vi "ELVIS III v1.1 Open SPI.vi"(7 "Allow multiple opens?":bool, 8 "error in (no error)":errorcluster, 10 "Channel Name":string, 11 "Resource name":T1 caption="RIO Device") -> (0 "error out":errorcluster, 2 "SPI Channel":T2, 3 "myRIO Ref Out":T3)   [LabVIEW 2021]
uses:
  <vilib>/myRIO/Common/Instrument Driver Framework/Utilities/typedefs/myRIO v1.0 Reference.ctl
  <vilib>/myRIO/Common/Instrument Driver Framework/Utilities/typedefs/Generic FPGA Reference.ctl
  <vilib>/myRIO/Common/Instrument Driver Framework/myRIO v1.0/SPI/typedefs/SPI Channels Enum.ctl
  <vilib>/userDefined/High Color/nirio_resource_hc.ctl
  <vilib>/myRIO/Common/Instrument Driver Framework/ELVIS III v1.0/SPI/typedefs/ELVIS III v1.0 SPI Channels Enum.ctl
  <vilib>/myRIO/Common/Instrument Driver Framework/ELVIS III v1.0/SPI/vis/ELVIS III v1.0 Build MUX Configuration SPI.vi
  <vilib>/myRIO/Common/Instrument Driver Framework/ELVIS III v1.0/Resource Manager/vis/ELVIS III v1.0 Create Configuration List.vi
  <vilib>/Utility/VariantDataType/GetNumericInfo.vi
  <vilib>/Utility/error.llb/Error Cluster From Error Code.vi
  <vilib>/myRIO/Common/Instrument Driver Framework/ELVIS III v1.0/Resource Manager/vis/ELVIS III v1.0 Reserve Channel List.vi
  <vilib>/myRIO/Common/Instrument Driver Framework/ELVIS III v1.0/Resource Manager/vis/ELVIS III v1.0 Configure IO.vi
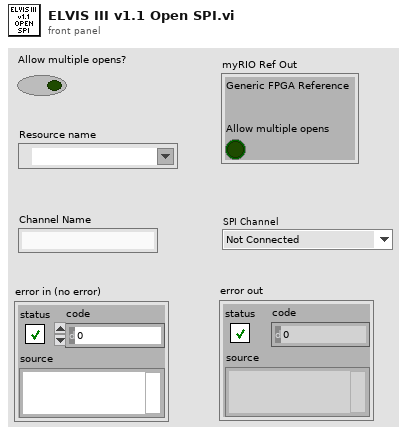
[diagram p1: front panel]
types:
  T1 = typedef "nirio_resource_hc.ctl" = tag
  T2 = typedef "SPI Channels Enum.ctl" = enum16{"Not Connected", "A/SPI", "B/SPI", "SPI/SPI"}
  T3 = typedef "myRIO v1.0 Reference.ctl" = cluster{"Generic FPGA Reference":T4, "Allow multiple opens":bool}
  T4 = typedef "Generic FPGA Reference.ctl" = refnum<k20>
  T5 = typedef "ELVIS III v1.0 SPI Channels Enum.ctl" = enum16{"Not Connected", "A/SPI", "B/SPI"}
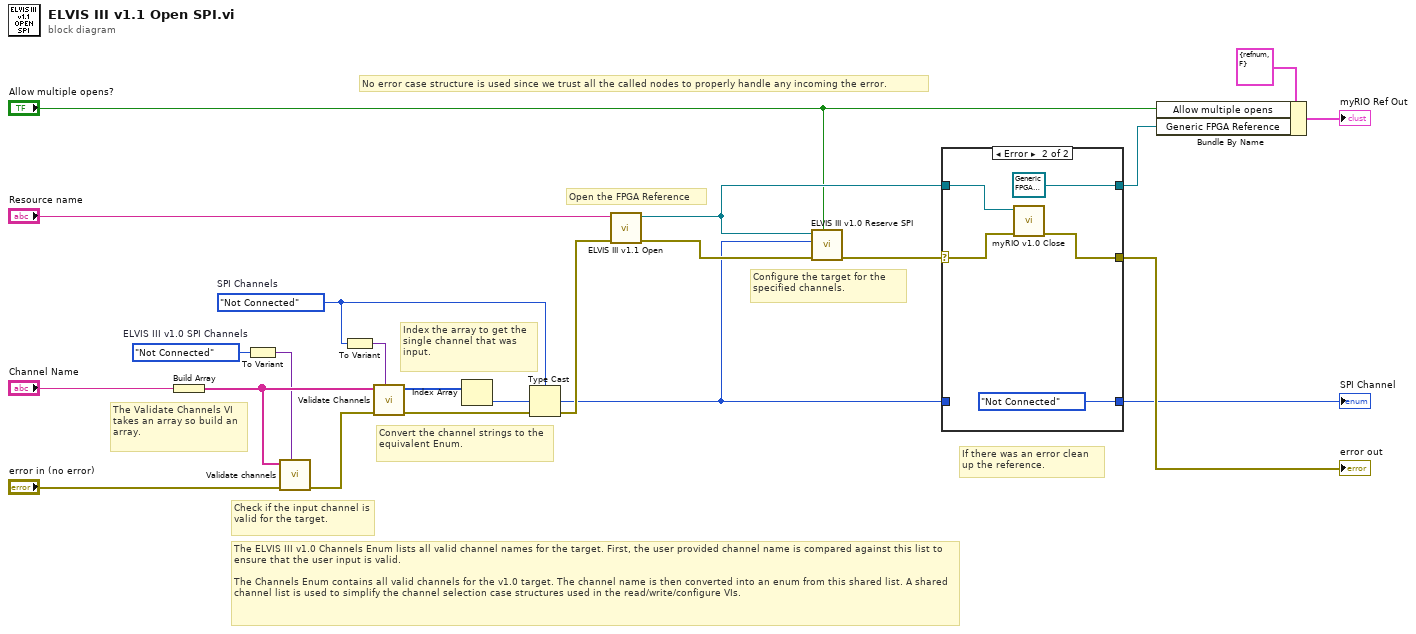
[diagram p0: block diagram]
diagram:
  w1 = SPI_Channels_Enum."Not Connected"  # SPI Channels
  w3 = ELVIS_III_v1.0_SPI_Channels_Enum."Not Connected"  # ELVIS III v1.0 SPI Channels
  # "The ELVIS III v1.0 Channels Enum lists all valid channel names for the target. First, the user provided channel name is compared against this list to ensure that the user input is valid.\n\nThe Channels Enum contains all valid channels for the v1.0 target. The channel name is then converted into an enum from this shared list. A shared channel list is used to simplify the channel selection case structures used in the read/write/configure VIs."
  # "Index the array to get the single channel that was input."
  # "The Validate Channels VI takes an array so build an array."
  # "If there was an error clean up the reference."
  # "Configure the target for the specified channels."
  # "Open the FPGA Reference"
  # "No error case structure is used since we trust all the called nodes to properly handle any incoming the error."
  # "Convert the channel strings to the equivalent Enum."
  # "Check if the input channel is valid for the target."
  n1 = Build Array("Channel Name") -> (w12:string[])
  n2 = To Variant(anything=w3) -> (Variant=w4:variant)
  n3 = call <vilib>:"Validate channels.vi"("Channels Enum Variant"=w4, "error in (no error)"="error in (no error)", "Channel Names"=w12) -> ("error out"=w21:errorcluster)  [unwired: 7 in, 1 out]
  n4 = To Variant(anything=w1) -> (Variant=w2:variant)
  n5 = call <vilib>:"Validate Channels.vi"("Channels Enum Variant"=w2, "error in (no error)"=w21, "Channel Names"=w12) -> ("error out"=w17:errorcluster, "Index Array"=w11:u16[])  [unwired: 7 in]
  n6 = Index Array(array=w11) -> (element=w10:u16)  [unwired: 1 in]
  n7 = Type Cast(type=w1, x=w10) -> (*(type *) &x=w9:T2)
  n8 = call <vilib>:"ELVIS III v1.1 Open.vi"("error in (no error)"=w17, "Resource name"="Resource name") -> ("error out"=w16:errorcluster, "myRIO FPGA Ref Out"=w14:T4)  [unwired: 8 in]
  n9 = call <vilib>:"ELVIS III v1.0 Reserve SPI.vi"("Allow multiple opens?"="Allow multiple opens?", "error in (no error)"=w16, "SPI Channel"=w9, "myRIO FPGA Ref In"=w14) -> ("error out"=w15:errorcluster)  [unwired: 7 in]
  n10 = case shown="Error" w15 {
    selector: w15 -> [w24 w30]
    tunnel: w14 -> [w25 w28]
    tunnel: [w25 T4 refnum ("myRIO FPGA Ref Out")] -> w19
    tunnel: [w24 w29] -> w18
    tunnel: w9 -> [w23 _]
    tunnel: [w23 SPI_Channels_Enum."Not Connected"] -> w8
    frame No Error {
    }
    frame Error {
      n11 = call <vilib>:"myRIO v1.0 Close.vi"("error in (no error)"=w30, "myRIO FPGA Ref In"=w28) -> ("error out"=w29:errorcluster)  [unwired: 9 in]
    }
  }
  "SPI Channel" <- w8
  "error out" <- w18
  n12 = Bundle By Name(cluster=T3 {"Generic FPGA Reference"=refnum, "Allow multiple opens"=FALSE} ("myRIO v1.0 Reference"), "Allow multiple opens"="Allow multiple opens?", "Generic FPGA Reference"=w19) -> (→"myRIO Ref Out":T3)
